vi "Teleop.vi"(10 "Match Info":T1={"Autonomous Elapsed Seconds"=0.0, "TeleOp Elapsed Seconds"=0.0, "Disabled Elapsed Seconds"=0.0, "Visited Autonomous"=FALSE, "Visited TeleOp"=FALSE, "Visited Disabled"=FALSE, "Autonomous Settings"={"Autonomous Style"=enum."Independent", "VI Refnum"=refnum}}, 11 "Call Context":T2) -> ()   [LabVIEW 2013]
doc: "This VI is called for each TeleOp packet received from the DS where the robot is not disabled. It is often used to read from the joysticks and update I/O or to update setpoints for timed control loops. It should complete and return within 20 milliseconds or it may miss DS packets."
uses:
  <vilib>/Rock Robotics/WPI/DriverStation/WPI_DriverStationDerivedRobotMode.ctl
  <vilib>/Rock Robotics/WPI/DriverStation/WPI_DriverStationMatch Info.ctl
  <vilib>/Rock Robotics/WPI/DriverStation/DriverStationLCD/WPI_DriverStationLCDLCDLine.ctl
  Robot Global Data.vi
  <vilib>/Rock Robotics/WPI/Joystick/WPI_JoystickGetSetRefNum.vi
  <vilib>/Rock Robotics/WPI/RobotDrive/WPI_RobotDriveGetSetRefNum.vi
  <vilib>/Rock Robotics/WPI/Solenoid/WPI_SolenoidSetEnum.vi
  <vilib>/Rock Robotics/WPI/Solenoid/WPI_SolenoidValue.ctl
panel:
  out "Numeric 1":dbl(slide) scale=0.0..100.0
  out "Boolean 2":bool
  out "Boolean 1":bool
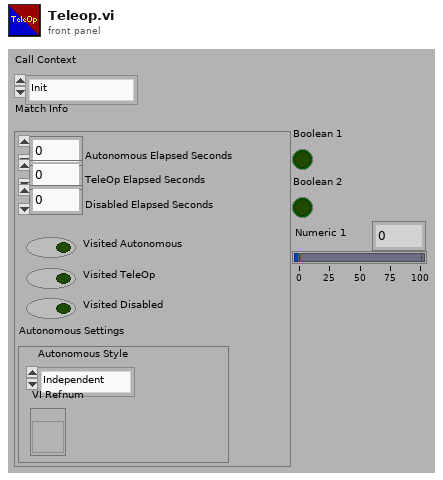
[diagram p1: front panel]
types:
  T1 = typedef "WPI_DriverStationMatch Info.ctl" = cluster{"Autonomous Elapsed Seconds":dbl, "TeleOp Elapsed Seconds":dbl, "Disabled Elapsed Seconds":dbl, "Visited Autonomous":bool, "Visited TeleOp":bool, "Visited Disabled":bool, "Autonomous Settings":cluster{"Autonomous Style":enum16{"Iterative", "Independent"}, "VI Refnum":refnum<vi>}}
  T2 = typedef "WPI_DriverStationDerivedRobotMode.ctl" = enum16{"Init", "Execute", "Stop"}
  T3 = typedef "WPI_DriverStationLCDLCDLine.ctl" = enum16{"Main - Line 1", "User - Line 2", "User - Line 3", "User - Line 4", "User - Line 5", "User - Line 6"}
  T4 = typedef "WPI_JoystickDevRef.ctl" = cluster{"Device":T5}
  T5 = typedef "WPI_JoystickDeviceEnum.ctl" = enum16{"USB 1", "USB 2", "USB 3", "USB 4", "Kinect 1", "Kinect 2"}
  T6 = typedef "WPI_JoystickButtonState.ctl" = cluster{"Button 1":bool, "Button 2":bool, "Button 3":bool, "Button 4":bool, "Button 5":bool, "Button 6":bool, "Button 7":bool, "Button 8":bool, "Button 9":bool, "Button 10":bool, "Button 11":bool, "Button 12":bool}
  T7 = cluster{"axis 1 (x)":dbl, "axis 2 (y)":dbl, "axis 3 (throttle)":dbl, "axis 4":dbl, "axis 5":dbl, "axis 6":dbl}
  T8 = typedef "WPI_SolenoidValue.ctl" = enum16{"Off", "On", "Forward", "Reverse"}
  T9 = typedef "WPI_SolenoidDevRef.ctl" = cluster{"DevStatus":errorcluster, "Solenoid Module":T10, "Forward Solenoid Channel":T11, "Reverse Solenoid Channel":T11}
  T10 = typedef "FPGA_TypedefSolenoidModule.ctl" = enum16{"Solenoid Module 1", "Solenoid Module 2"}
  T11 = typedef "WPI_SolenoidChannel.ctl" = enum8{"Solenoid 1", "Solenoid 2", "Solenoid 3", "Solenoid 4", "Solenoid 5", "Solenoid 6", "Solenoid 7", "Solenoid 8", "Invalid"}
  T12 = typedef "WPI_RobotDriveDevRef.ctl" = cluster{"DevStatus":errorcluster, "Motors[]":T13[], "Square Inputs":bool, "Max Output":dbl, "Isochronous":bool}
  T13 = typedef "WPI_MotorControlDeviceRef.ctl" = cluster{"DeviceStatus":errorcluster, "Type":enum16{"PWM", "CAN"}, "PWM":cluster{"Digital Module":T14, "PWM Channel":T15, "DeadBand":T16}, "CAN":cluster{"Device Number":u8, "Control Mode":T17, "Semaphore":T18, "Max Vout":dbl}, "Invert":bool, "TransformRef":T19, "InvTransformRef":T19}
  T14 = typedef "FPGA_TypedefDigitalModule.ctl" = enum16{"Digital Module 1", "Digital Module 2"}
  T15 = typedef "FPGA_DIOPWMChannel.ctl" = enum8{"PWM 1", "PWM 2", "PWM 3", "PWM 4", "PWM 5", "PWM 6", "PWM 7", "PWM 8", "PWM 9", "PWM 10", "Invalid"}
  T16 = typedef "WPI_PWMDeadband.ctl" = cluster{"Name":string, "maxPositivePwm":i32, "minPositivePwm":i32, "centerPwm":i32, "maxNegativePwm":i32, "minNegativePwm":i32, "angularRange":u16}
  T17 = typedef "WPI_CANJaguar_ControlMode.ctl" = enum8{"Percent VBus", "Current", "Speed", "Position", "Voltage"}
  T18 = typedef "Semaphore RefNum" = refnum<k1>
  T19 = typedef "WPI_PWMTransform_ConPane.ctl" = refnum<vi>
  T20 = enum16{"Reset", "Start", "Reset 2", "Manual", "Get ready to Fire", "Disengage Gearbox", "Ready to Fire", "Firing", "Firing Completed", "Reengage Gearbox"}
  T21 = typedef "WPI_AnalogChannelDevRef.ctl" = cluster{"DevStatus":errorcluster, "Analog Module":T22, "Analog Channel":T23}
  T22 = typedef "FPGA_TypedefAnalogModule.ctl" = enum16{"Analog Module 1", "Analog Module 2"}
  T23 = typedef "FPGA_AIChannel.ctl" = enum8{"AI 1", "AI 2", "AI 3", "AI 4", "AI 5", "AI 6", "AI 7", "AI 8", "Invalid"}
  T24 = typedef "WPI_DigitalInputDevRef.ctl" = cluster{"DevStatus":errorcluster, "DIO Channel":T25, "Digital Module":T14}
  T25 = typedef "FPGA_DIOChannel.ctl" = enum8{"DIO 1", "DIO 2", "DIO 3", "DIO 4", "DIO 5", "DIO 6", "DIO 7", "DIO 8", "DIO 9", "DIO 10", "DIO 11", "DIO 12", "DIO 13", "DIO 14", "Invalid"}
  T26 = typedef "WPI_RelayDevRef.ctl" = cluster{"DevStatus":errorcluster, "Relay Channel":T27, "Digital Module":T14, "Relay Direction":T28}
  T27 = typedef "FPGA_DIORelayChannel.ctl" = enum8{"Relay 1", "Relay 2", "Relay 3", "Relay 4", "Relay 5", "Relay 6", "Relay 7", "Relay 8", "Invalid"}
  T28 = typedef "WPI_RelayDirection.ctl" = enum16{"Both directions", "Forward only", "Reverse only"}
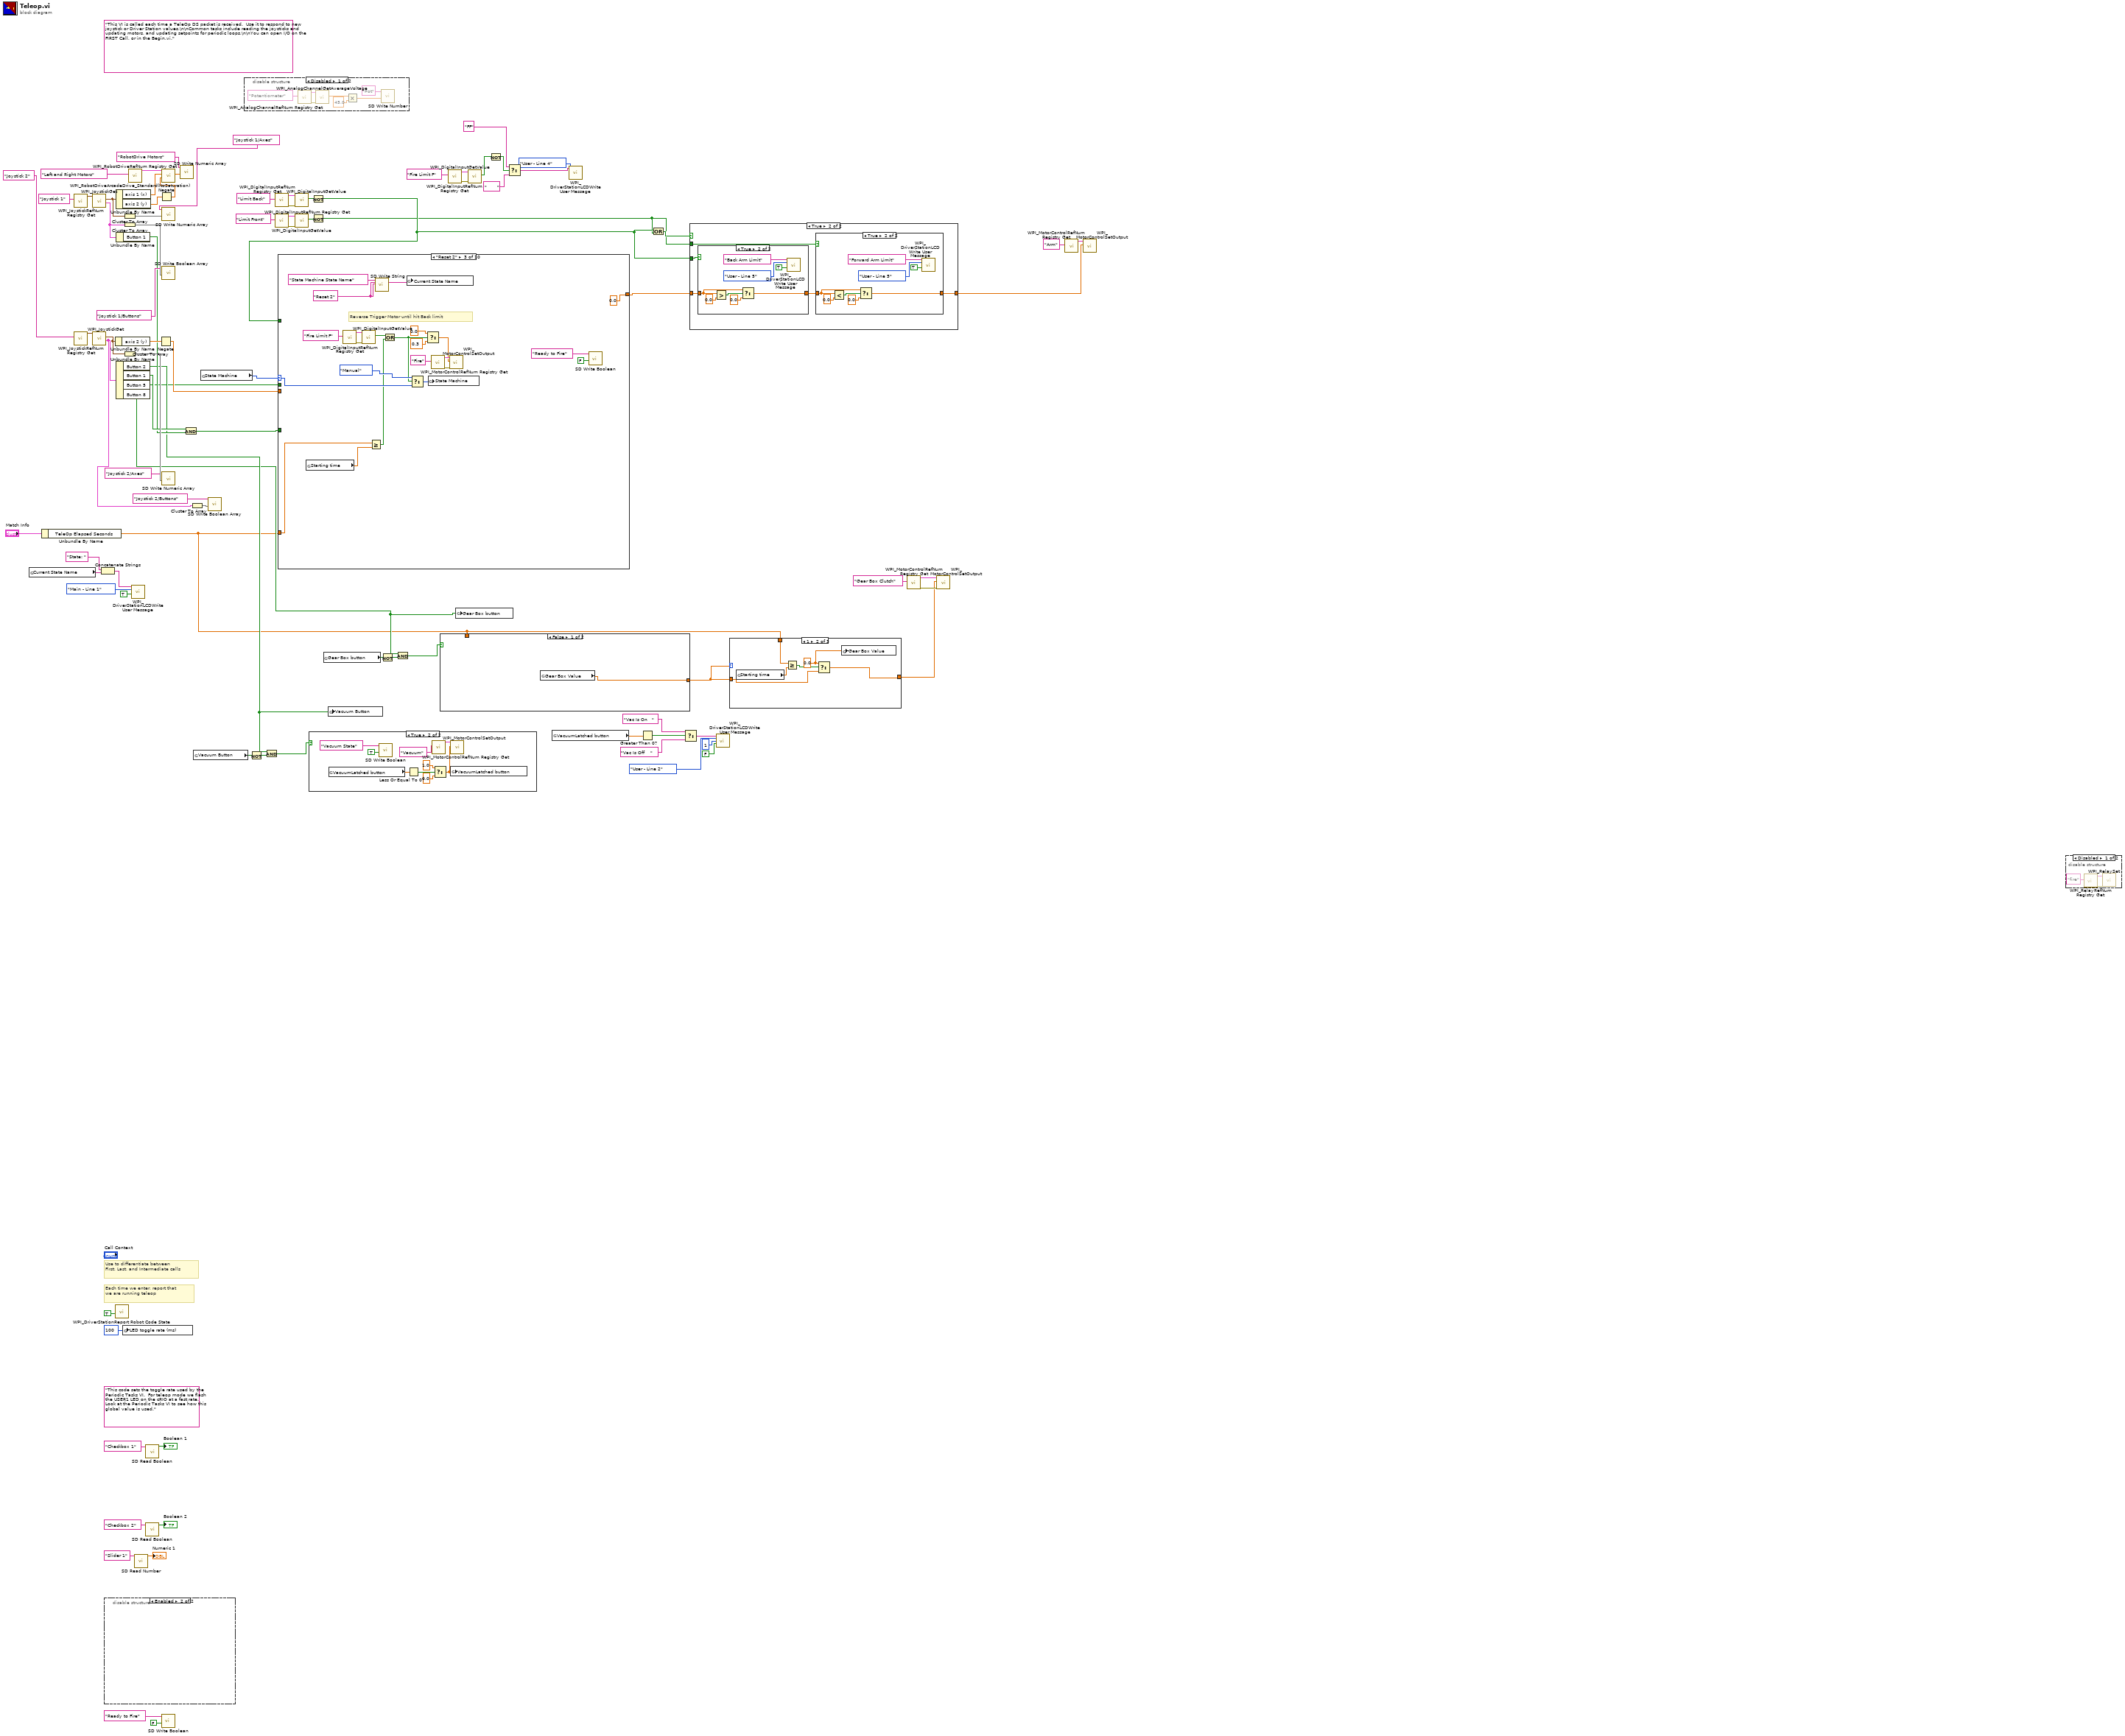
[diagram p0: block diagram]
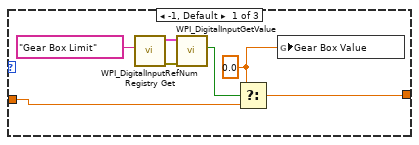
[diagram p2: hidden frame]
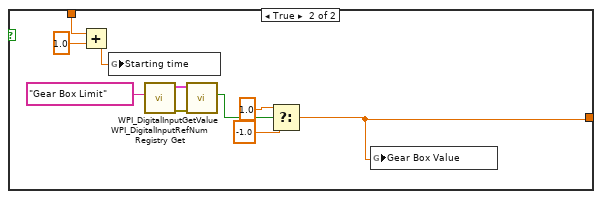
[diagram p4: hidden frame]
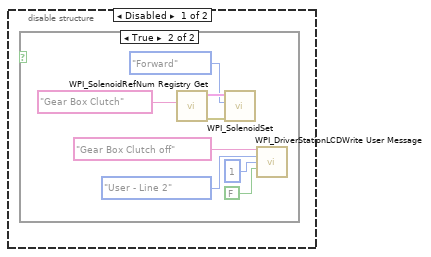
[diagram p11: hidden frame]
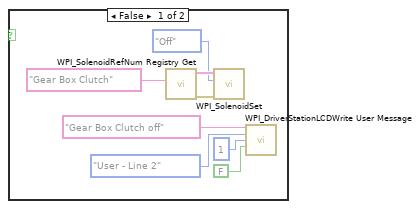
[diagram p12: hidden frame]
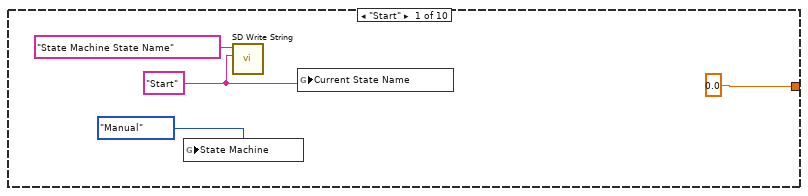
[diagram p13: hidden frame]
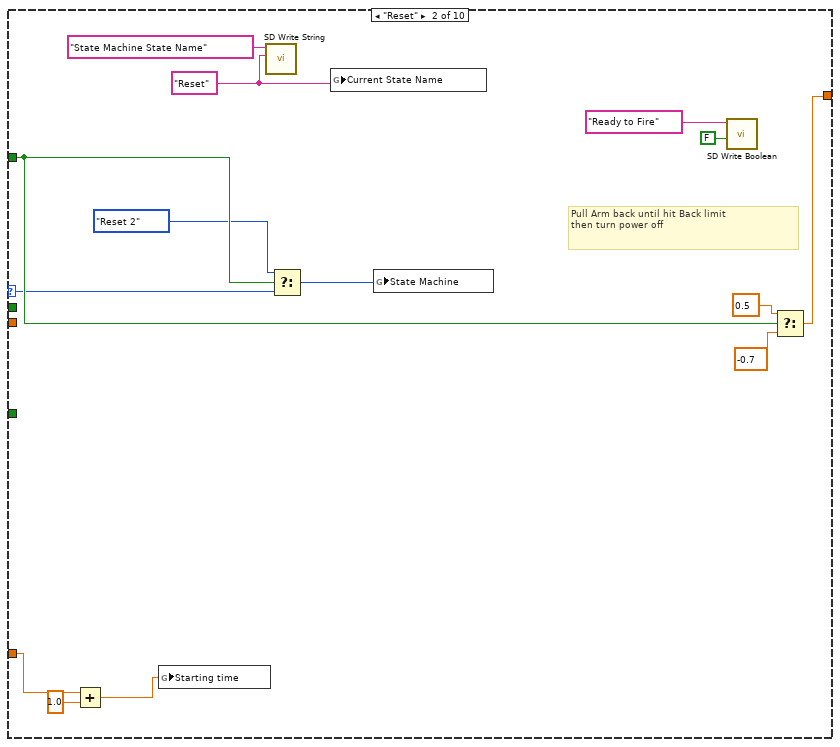
[diagram p14: hidden frame]
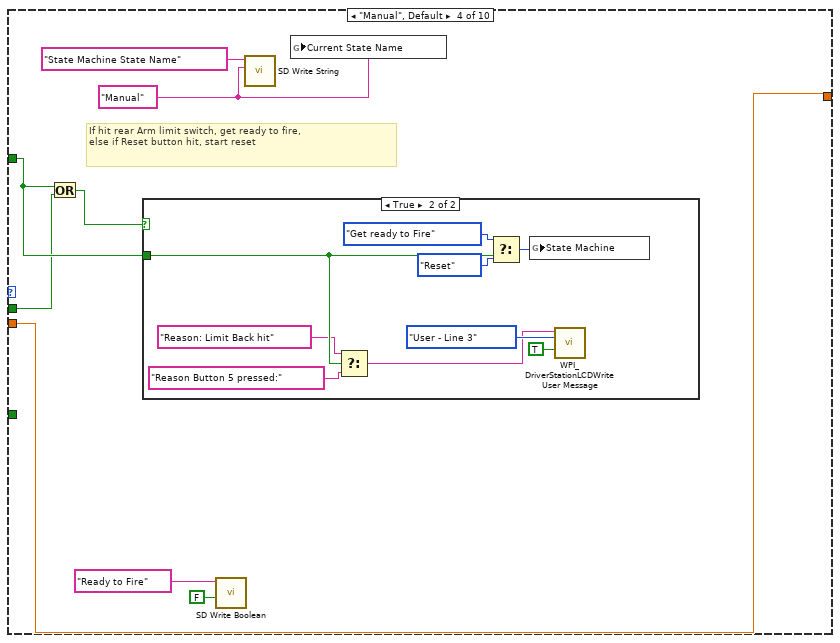
[diagram p15: hidden frame]
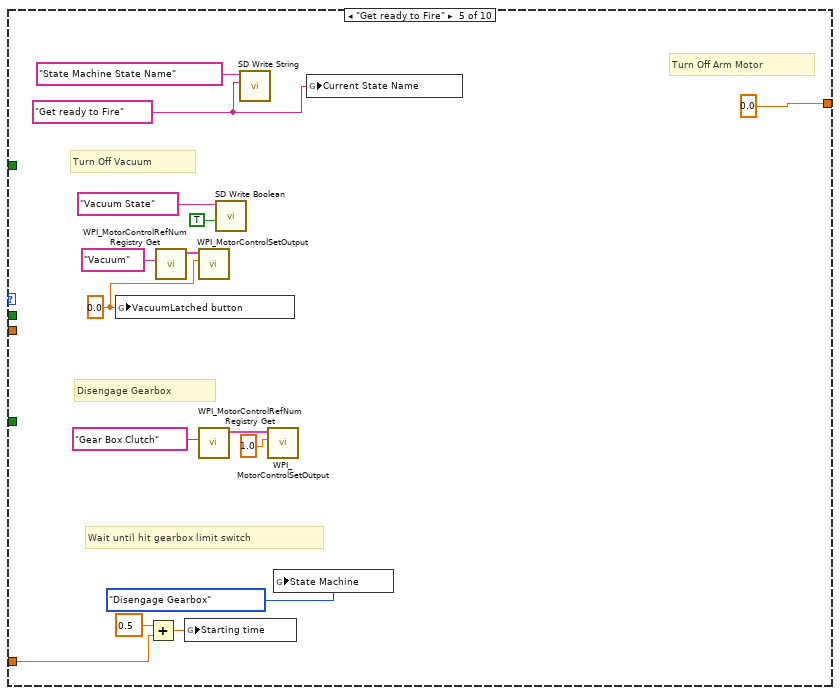
[diagram p17: hidden frame]
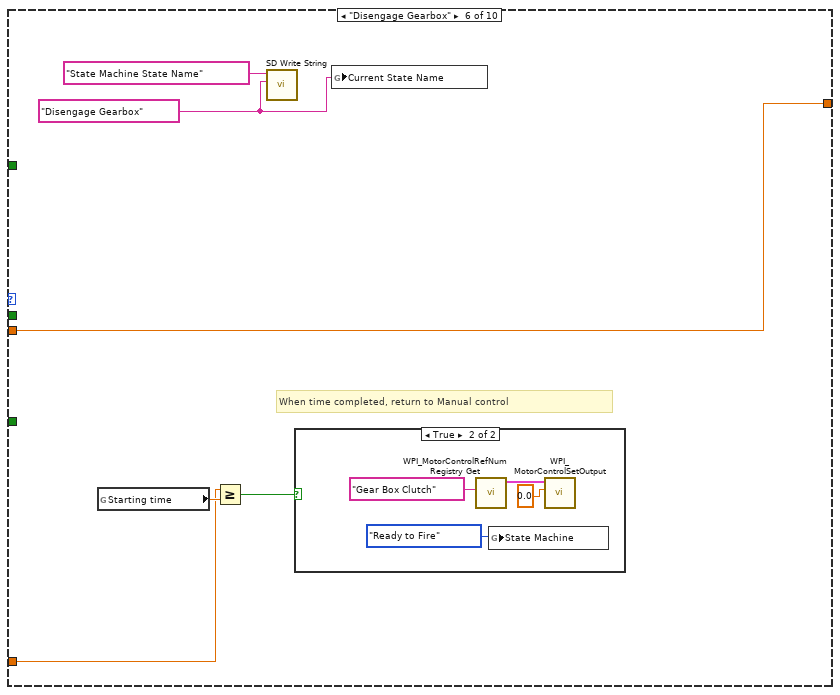
[diagram p18: hidden frame]
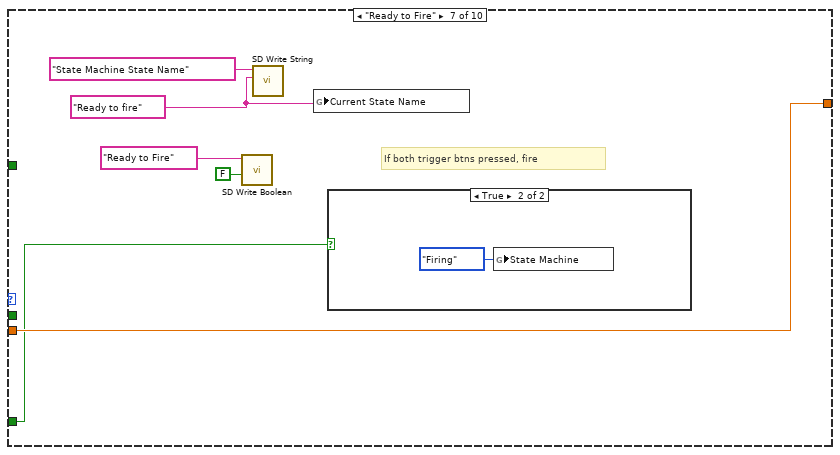
[diagram p20: hidden frame]
diagram:
  (unwired) "This code sets the toggle rate used by the Periodic Tasks VI.  For teleop mode we flash the USER1 LED on the cRIO at a fast rate.  Look at the Periodic Tasks VI to see how this global value is used."
  (unwired) "This VI is called each time a TeleOp DS packet is received.  Use it to respond to new joystick or Driver Station values.\n\nCommon tasks include reading the joysticks and updating motors, and updating setpoints for periodic loops.\n\nYou can open I/O on the FIRST Call, or in the Begin.vi."
  # "Each time we enter, report that\nwe are running teleop"
  # "Use to differentiate between\nFirst, Last, and Intermediate calls"
  n1 = global read "Robot Global Data.vi" "Current State Name"() -> (w23:string)
  n2 = Unbundle By Name("Match Info") -> ("TeleOp Elapsed Seconds"=w1:dbl)
  n3 = call <vilib>:"WPI_JoystickRefNum Registry Get.vi"("refnum name"="Joystick 1") -> ("JoystickDevRef"=w87:T4)  [unwired: 1 in, 9 out]
  n4 = call <vilib>:"WPI_JoystickRefNum Registry Get.vi"("refnum name"="Joystick 2") -> ("JoystickDevRef"=w70:T4)  [unwired: 1 in, 9 out]
  n5 = call <vilib>:"WPI_JoystickGet.vi"("JoystickDevRef"=w87) -> ("Buttons"=w62:T6, "Axes"=w82:T7)  [unwired: 1 in, 4 out]
  n6 = call <vilib>:"WPI_JoystickGet.vi"("JoystickDevRef"=w70) -> ("Buttons"=w64:T6, "Axes"=w67:T7)  [unwired: 1 in, 4 out]
  n7 = Concatenate Strings("State: " ("line text"), w23) -> (w22:string)
  n8 = disable-structure shown="Enabled" {
    frame Disabled {
      n9 = case shown="True" {
        selector: _ -> [_ _]
        frame False {
          n10 = call <vilib>:"WPI_SolenoidRefNum Registry Get.vi"("refnum name"="Gear Box Clutch") -> ("error out"=w98:errorcluster, "SolenoidDevRef"=w99:T9)  [unwired: 9 in]
          n11 = call-poly <vilib>:"WPI_SolenoidSet.vi"("error in (no error)"=w98, "Value"=WPI_SolenoidValue."Off", "SolenoidDevRef"=w99) -> ()  [unwired: 7 in, 2 out]
          n12 = call <vilib>:"WPI_DriverStationLCDWrite User Message.vi"("line text"="Gear Box Clutch off", "line"=WPI_DriverStationLCDLCDLine."User - Line 2", "starting column"=i8 1, "clear line before write (T)"=FALSE) -> ()  [unwired: 11 in, 1 out]
        }
        frame True {
          n13 = call <vilib>:"WPI_SolenoidRefNum Registry Get.vi"("refnum name"="Gear Box Clutch") -> ("error out"=w106:errorcluster, "SolenoidDevRef"=w107:T9)  [unwired: 9 in]
          n14 = call-poly <vilib>:"WPI_SolenoidSet.vi"("error in (no error)"=w106, "Value"=WPI_SolenoidValue."Forward", "SolenoidDevRef"=w107) -> ()  [unwired: 7 in, 2 out]
          n15 = call <vilib>:"WPI_DriverStationLCDWrite User Message.vi"("line text"="Gear Box Clutch off", "line"=WPI_DriverStationLCDLCDLine."User - Line 2", "starting column"=i8 1, "clear line before write (T)"=FALSE) -> ()  [unwired: 11 in, 1 out]
        }
      }
    }
    frame Enabled {
    }
  }
  n16 = Unbundle By Name(w67) -> ("axis 2 (y)"=w63:dbl)
  n17 = call <vilib>:"WPI_DriverStationReport Robot Code State.vi"("TeleOp"=TRUE ("Autonomous")) -> ()  [unwired: 10 in, 1 out]
  n18 = Unbundle By Name(w82) -> ("axis 1 (x)"=w89:dbl, "axis 2 (y)"=w12:dbl)
  n19 = Unbundle By Name(w62) -> ("Button 1"=w60:bool)
  n20 = Unbundle By Name(w64) -> ("Button 2"=w45:bool, "Button 1"=w61:bool, "Button 5"=w27:bool, "Button 8"=w4:bool)
  n21 = global write "Robot Global Data.vi" "LED toggle rate (ms)"(u32 100 ("LED ms toggle rate")) -> ()
  n22 = Cluster To Array(cluster=w82) -> (array=w81:dbl[])
  n23 = Cluster To Array(cluster=w62) -> (array=w84:bool[])
  n24 = Cluster To Array(cluster=w67) -> (array=w66:dbl[])
  n25 = call <vilib>:"WPI_RobotDriveRefNum Registry Get.vi"("refnum name"="Left and Right Motors") -> ("RobotDriveDevRef"=w90:T12)  [unwired: 1 in, 9 out]
  n26 = call <vilib>:"WPI_DriverStationLCDWrite User Message.vi"("line text"=w22, "line"=WPI_DriverStationLCDLCDLine."Main - Line 1", "clear line before write (T)"=TRUE) -> ()  [unwired: 12 in, 1 out]
  n27 = call <vilib>:"SD Read Number.vi"("Name"="Slider 1" ("refnum name")) -> ("Numeric"=→"Numeric 1":dbl)  [unwired: 8 in, 2 out]
  n28 = call <vilib>:"SD Read Boolean.vi"("Name"="Checkbox 1" ("refnum name")) -> ("Boolean"=→"Boolean 1":bool)  [unwired: 8 in, 2 out]
  n29 = call <vilib>:"SD Read Boolean.vi"("Name"="Checkbox 2" ("refnum name")) -> ("Boolean"=→"Boolean 2":bool)  [unwired: 8 in, 2 out]
  n30 = Negate(x=w63) -> (-x=w48:dbl)
  n31 = Negate(x=w12) -> (-x=w11:dbl)
  n32 = call <vilib>:"SD Write Boolean.vi"("Boolean"=FALSE, "Name"="Ready to Fire") -> ()  [unwired: 8 in, 2 out]
  n33 = call <vilib>:"WPI_RobotDriveArcadeDrive_Standard(NoSaturation).vi"("Y axis value"=w11, "X axis value"=w89, "RobotDriveDevRef"=w90) -> ("Motor Values"=w78:dbl[])  [unwired: 1 in, 7 out]
  n34 = call <vilib>:"SD Write Numeric Array.vi"("Numeric Array"=w81, "Name"="Joystick 1/Axes") -> ()  [unwired: 8 in, 2 out]
  n35 = call <vilib>:"SD Write Boolean Array.vi"("Boolean Array"=w84, "Name"="Joystick 1/Buttons") -> ()  [unwired: 8 in, 2 out]
  n36 = call <vilib>:"SD Write Numeric Array.vi"("Numeric Array"=w66, "Name"="Joystick 2/Axes") -> ()  [unwired: 8 in, 2 out]
  n37 = call <vilib>:"SD Write Numeric Array.vi"("Numeric Array"=w78, "Name"="RobotDrive Motors") -> ()  [unwired: 8 in, 2 out]
  n38 = And(x=w61, y=w60) -> (x .and. y?=w43:bool)
  n39 = Cluster To Array(cluster=w64) -> (array=w69:bool[])
  n40 = global read "Robot Global Data.vi" "Vacuum Button"() -> (w46:bool)
  n41 = global read "Robot Global Data.vi" "State Machine"() -> (w44:T20)
  n42 = call <vilib>:"SD Write Boolean Array.vi"("Boolean Array"=w69, "Name"="Joystick 2/Buttons") -> ()  [unwired: 8 in, 2 out]
  n43 = disable-structure shown="Disabled" {
    frame Disabled {
      n44 = call <vilib>:"WPI_AnalogChannelRefNum Registry Get.vi"("refnum name"="Potentiometer") -> ("error out"=w115:errorcluster, "AIDeviceRef"=w114:T21)  [unwired: 9 in]
      n45 = call <vilib>:"WPI_AnalogChannelGetAverageVoltage.vi"("error in (no error)"=w115, "AIDeviceRef"=w114) -> ("Voltage"=w110:dbl)  [unwired: 7 in, 2 out]
      n46 = Multiply(x=w110, y=45.0) -> (x*y=w109:dbl)
      n47 = call <vilib>:"SD Write Number.vi"("Numeric"=w109, "Name"="Pot") -> ()  [unwired: 8 in, 2 out]
    }
    frame Enabled {
    }
  }
  n48 = Not(x=w46) -> (.not. x?=w47:bool)
  n49 = And(x=w45, y=w47) -> (x .and. y?=w37:bool)
  n50 = call <vilib>:"WPI_DigitalInputRefNum Registry Get.vi"("refnum name"="Limit Back") -> ("error out"=w54:errorcluster, "DigitalInputDevRef"=w53:T24)  [unwired: 9 in]
  n51 = call <vilib>:"WPI_DigitalInputRefNum Registry Get.vi"("refnum name"="Limit Front") -> ("error out"=w51:errorcluster, "DigitalInputDevRef"=w52:T24)  [unwired: 9 in]
  n52 = call <vilib>:"WPI_DigitalInputGetValue.vi"("error in (no error)"=w54, "DigitalInputDevRef"=w53) -> ("Value"=w42:bool)  [unwired: 7 in, 2 out]
  n53 = call <vilib>:"WPI_DigitalInputGetValue.vi"("error in (no error)"=w51, "DigitalInputDevRef"=w52) -> ("Value"=w40:bool)  [unwired: 7 in, 2 out]
  n54 = case shown="True" w37 {
    frame False {
    }
    frame True {
      n55 = global read "Robot Global Data.vi" "VacuumLatched button"() -> (w122:dbl)
      n56 = call <vilib>:"SD Write Boolean.vi"("Boolean"=TRUE, "Name"="Vacuum State") -> ()  [unwired: 8 in, 2 out]
      n57 = Less Or Equal To 0?(x=w122) -> (x <= 0?=w117:bool)
      n58 = call <vilib>:"WPI_MotorControlRefNum Registry Get.vi"("refnum name"="Vacuum") -> ("MotorControlDevRef"=w119:T13)  [unwired: 9 in, 1 out]
      n59 = Select(t=1.0 ("Numeric"), s=w117, f=0.0) -> (s? t:f=w118:dbl)
      n60 = call <vilib>:"WPI_MotorControlSetOutput.vi"("Output"=w118, "MotorControlDevRef"=w119) -> ()  [unwired: 7 in, 3 out]
      n61 = global write "Robot Global Data.vi" "VacuumLatched button"(w118) -> ()
    }
  }
  n62 = Not(x=w42) -> (.not. x?=w41:bool)
  n63 = case shown="\"Reset 2\"" w44 {
    selector: w44 -> [_ w136 w157 _ _ _ _ w218 _ _]
    tunnel: w48 -> [_ _ _ w166 _ w202 w212 w230 w239 w246]
    tunnel: [0.0 w137 0.0 w166 0.0 w202 w212 w230 w239 w246] -> w38
    tunnel: w43 -> [_ _ _ _ _ _ w208 _ _ _]
    tunnel: w41 -> [_ w140 _ w168 _ _ _ _ _ _]
    tunnel: w1 -> [_ w131 w146 _ w183 w197 _ _ _ _]
    tunnel: w27 -> [_ _ _ w165 _ _ _ _ _ _]
    frame "Start" {
      w126 = "Start" ("line text")
      n64 = global write "Robot Global Data.vi" "State Machine"(T20."Manual" ("State Machine")) -> ()
      n65 = call <vilib>:"SD Write String.vi"("Table Prefix"=w126, "Name"="State Machine State Name") -> ()  [unwired: 8 in, 2 out]
      n66 = global write "Robot Global Data.vi" "Current State Name"(w126) -> ()
    }
    frame "Reset" {
      w134 = "Reset" ("line text")
      # "Pull Arm back until hit Back limit\nthen turn power off"
      n67 = Add(x=w131, y=1.0) -> (x+y=w129:dbl)
      n68 = global write "Robot Global Data.vi" "Starting time"(w129) -> ()
      n69 = call <vilib>:"SD Write String.vi"("Table Prefix"=w134, "Name"="State Machine State Name") -> ()  [unwired: 8 in, 2 out]
      n70 = Select(t=T20."Reset 2" ("s? t:f"), s=w140, f=w136) -> (s? t:f=w133:T20)
      n71 = global write "Robot Global Data.vi" "Current State Name"(w134) -> ()
      n72 = global write "Robot Global Data.vi" "State Machine"(w133) -> ()
      n73 = call <vilib>:"SD Write Boolean.vi"("Boolean"=FALSE, "Name"="Ready to Fire") -> ()  [unwired: 8 in, 2 out]
      n74 = Select(t=0.5, s=w140, f=-0.7) -> (s? t:f=w137:dbl)
    }
    frame "Reset 2" {
      w149 = "Reset 2" ("line text")
      # "Reverse Trigger Motor until hit Back limit"
      n75 = global read "Robot Global Data.vi" "Starting time"() -> (w145:dbl)
      n76 = call <vilib>:"WPI_DigitalInputRefNum Registry Get.vi"("refnum name"="Fire Limit F") -> ("error out"=w154:errorcluster, "DigitalInputDevRef"=w153:T24)  [unwired: 9 in]
      n77 = call <vilib>:"WPI_DigitalInputGetValue.vi"("error in (no error)"=w154, "DigitalInputDevRef"=w153) -> ("Value"=w147:bool)  [unwired: 7 in, 2 out]
      n78 = Greater Or Equal?(x=w146, y=w145) -> (x >= y?=w144:bool)
      n79 = call <vilib>:"SD Write String.vi"("Table Prefix"=w149, "Name"="State Machine State Name") -> ()  [unwired: 8 in, 2 out]
      n80 = Or(x=w147, y=w144) -> (x .or. y?=w143:bool)
      n81 = global write "Robot Global Data.vi" "Current State Name"(w149) -> ()
      n82 = Select(t=T20."Manual" ("s? t:f"), s=w143, f=w157) -> (s? t:f=w156:T20)
      n83 = Select(t=0.0, s=w143, f=0.3) -> (s? t:f=w151:dbl)
      n84 = global write "Robot Global Data.vi" "State Machine"(w156) -> ()
      n85 = call <vilib>:"WPI_MotorControlRefNum Registry Get.vi"("refnum name"="Fire") -> ("error out"=w162:errorcluster, "MotorControlDevRef"=w161:T13)  [unwired: 9 in]
      n86 = call <vilib>:"WPI_MotorControlSetOutput.vi"("error in (no error)"=w162, "Output"=w151, "MotorControlDevRef"=w161) -> ()  [unwired: 6 in, 3 out]
      n87 = call <vilib>:"SD Write Boolean.vi"("Boolean"=FALSE, "Name"="Ready to Fire") -> ()  [unwired: 8 in, 2 out]
    }
    frame "Manual", Default {
      w167 = "Manual" ("line text")
      # "If hit rear Arm limit switch, get ready to fire, \nelse if Reset button hit, start reset"
      n88 = Or(x=w168, y=w165) -> (x .or. y?=w169:bool)
      n89 = case shown="True" w169 {
        tunnel: w168 -> [_ w178]
        frame False {
        }
        frame True {
          n90 = Select(t="Reason: Limit Back hit" ("line text"), s=w178, f="Reason Button 5 pressed:" ("line text")) -> (s? t:f=w173:string)
          n91 = Select(t=T20."Get ready to Fire" ("State Machine"), s=w178, f=T20."Reset" ("State Machine")) -> (s? t:f=w180:T20)
          n92 = global write "Robot Global Data.vi" "State Machine"(w180) -> ()
          n93 = call <vilib>:"WPI_DriverStationLCDWrite User Message.vi"("line text"=w173, "line"=WPI_DriverStationLCDLCDLine."User - Line 3", "clear line before write (T)"=TRUE) -> ()  [unwired: 12 in, 1 out]
        }
      }
      n94 = call <vilib>:"SD Write Boolean.vi"("Boolean"=FALSE, "Name"="Ready to Fire") -> ()  [unwired: 8 in, 2 out]
      n95 = call <vilib>:"SD Write String.vi"("Table Prefix"=w167, "Name"="State Machine State Name") -> ()  [unwired: 8 in, 2 out]
      n96 = global write "Robot Global Data.vi" "Current State Name"(w167) -> ()
    }
    frame "Get ready to Fire" {
      w186 = "Get ready to Fire" ("line text")
      w192 = 0.0 ("f")
      # "Wait until hit gearbox limit switch"
      # "Disengage Gearbox"
      # "Turn Off Arm Motor"
      # "Turn Off Vacuum"
      n97 = global write "Robot Global Data.vi" "VacuumLatched button"(w192) -> ()
      n98 = Add(x=0.5 ("Starting time"), y=w183) -> (x+y=w184:dbl)
      n99 = call <vilib>:"WPI_MotorControlRefNum Registry Get.vi"("refnum name"="Vacuum") -> ("MotorControlDevRef"=w193:T13)  [unwired: 9 in, 1 out]
      n100 = global write "Robot Global Data.vi" "Starting time"(w184) -> ()
      n101 = call <vilib>:"WPI_MotorControlSetOutput.vi"("Output"=w192, "MotorControlDevRef"=w193) -> ()  [unwired: 7 in, 3 out]
      n102 = call <vilib>:"WPI_MotorControlRefNum Registry Get.vi"("refnum name"="Gear Box Clutch") -> ("MotorControlDevRef"=w191:T13)  [unwired: 9 in, 1 out]
      n103 = call <vilib>:"SD Write Boolean.vi"("Boolean"=TRUE, "Name"="Vacuum State") -> ()  [unwired: 8 in, 2 out]
      n104 = call <vilib>:"SD Write String.vi"("Table Prefix"=w186, "Name"="State Machine State Name") -> ()  [unwired: 8 in, 2 out]
      n105 = call <vilib>:"WPI_MotorControlSetOutput.vi"("Output"=1.0 ("Numeric"), "MotorControlDevRef"=w191) -> ()  [unwired: 7 in, 3 out]
      n106 = global write "Robot Global Data.vi" "State Machine"(T20."Disengage Gearbox" ("State Machine")) -> ()
      n107 = global write "Robot Global Data.vi" "Current State Name"(w186) -> ()
    }
    frame "Disengage Gearbox" {
      w200 = "Disengage Gearbox" ("line text")
      # "When time completed, return to Manual control"
      n108 = global read "Robot Global Data.vi" "Starting time"() -> (w199:dbl)
      n109 = Greater Or Equal?(x=w197, y=w199) -> (x >= y?=w198:bool)
      n110 = call <vilib>:"SD Write String.vi"("Table Prefix"=w200, "Name"="State Machine State Name") -> ()  [unwired: 8 in, 2 out]
      n111 = case shown="True" w198 {
        frame False {
        }
        frame True {
          n112 = call <vilib>:"WPI_MotorControlRefNum Registry Get.vi"("refnum name"="Gear Box Clutch") -> ("MotorControlDevRef"=w206:T13)  [unwired: 9 in, 1 out]
          n113 = global write "Robot Global Data.vi" "State Machine"(T20."Ready to Fire" ("State Machine")) -> ()
          n114 = call <vilib>:"WPI_MotorControlSetOutput.vi"("Output"=0.0 ("Numeric"), "MotorControlDevRef"=w206) -> ()  [unwired: 7 in, 3 out]
        }
      }
      n115 = global write "Robot Global Data.vi" "Current State Name"(w200) -> ()
    }
    frame "Ready to Fire" {
      w207 = "Ready to fire" ("line text")
      # "If both trigger btns pressed, fire"
      n116 = call <vilib>:"SD Write Boolean.vi"("Boolean"=FALSE, "Name"="Ready to Fire") -> ()  [unwired: 8 in, 2 out]
      n117 = call <vilib>:"SD Write String.vi"("Table Prefix"=w207, "Name"="State Machine State Name") -> ()  [unwired: 8 in, 2 out]
      n118 = global write "Robot Global Data.vi" "Current State Name"(w207) -> ()
      n119 = case shown="True" w208 {
        frame False {
        }
        frame True {
          n120 = global write "Robot Global Data.vi" "State Machine"(T20."Firing" ("State Machine")) -> ()
        }
      }
    }
    frame "Firing" {
      w215 = "Firing" ("line text")
      # "Run Trigger motor forward until hit forward limit"
      n121 = call <vilib>:"WPI_DigitalInputRefNum Registry Get.vi"("refnum name"="Fire Limit F") -> ("error out"=w221:errorcluster, "DigitalInputDevRef"=w222:T24)  [unwired: 9 in]
      n122 = call <vilib>:"WPI_DigitalInputGetValue.vi"("error in (no error)"=w221, "DigitalInputDevRef"=w222) -> ("Value"=w220:bool)  [unwired: 7 in, 2 out]
      n123 = Not(x=w220) -> (.not. x?=w217:bool)
      n124 = call <vilib>:"SD Write String.vi"("Table Prefix"=w215, "Name"="State Machine State Name") -> ()  [unwired: 8 in, 2 out]
      n125 = Select(t=T20."Firing Completed" ("s? t:f"), s=w217, f=w218) -> (s? t:f=w216:T20)
      n126 = global write "Robot Global Data.vi" "Current State Name"(w215) -> ()
      n127 = global write "Robot Global Data.vi" "State Machine"(w216) -> ()
      n128 = Select(t=0.0, s=w217, f=-0.8) -> (s? t:f=w224:dbl)
      n129 = call <vilib>:"WPI_MotorControlRefNum Registry Get.vi"("refnum name"="Fire") -> ("error out"=w229:errorcluster, "MotorControlDevRef"=w228:T13)  [unwired: 9 in]
      n130 = call <vilib>:"WPI_MotorControlSetOutput.vi"("error in (no error)"=w229, "Output"=w224, "MotorControlDevRef"=w228) -> ()  [unwired: 6 in, 3 out]
    }
    frame "Firing Completed" {
      w232 = "Firing Completed" ("line text")
      # "Run for .5 secs"
      # "Re-engage Gearbox by running clutch motor in reverse"
      # "Turn off Trigger motor"
      n131 = call <vilib>:"WPI_MotorControlRefNum Registry Get.vi"("refnum name"="Fire") -> ("error out"=w238:errorcluster, "MotorControlDevRef"=w237:T13)  [unwired: 9 in]
      n132 = call <vilib>:"WPI_MotorControlSetOutput.vi"("error in (no error)"=w238, "Output"=0.0, "MotorControlDevRef"=w237) -> ()  [unwired: 6 in, 3 out]
      n133 = call <vilib>:"SD Write String.vi"("Table Prefix"=w232, "Name"="State Machine State Name") -> ()  [unwired: 8 in, 2 out]
      n134 = global write "Robot Global Data.vi" "State Machine"(T20."Reengage Gearbox" ("State Machine")) -> ()
      n135 = global write "Robot Global Data.vi" "Gear Box Value"(-1.0 ("Numeric")) -> ()
      n136 = global write "Robot Global Data.vi" "Current State Name"(w232) -> ()
    }
    frame "Reengage Gearbox" {
      w244 = "Reengage Gearbox" ("line text")
      # "Keep moving gearbox motor until hit limit switch"
      n137 = call <vilib>:"WPI_DigitalInputRefNum Registry Get.vi"("refnum name"="Gear Box Limit") -> ("error out"=w242:errorcluster, "DigitalInputDevRef"=w243:T24)  [unwired: 9 in]
      n138 = call <vilib>:"WPI_DigitalInputGetValue.vi"("error in (no error)"=w242, "DigitalInputDevRef"=w243) -> ("Value"=w240:bool)  [unwired: 7 in, 2 out]
      n139 = call <vilib>:"SD Write String.vi"("Table Prefix"=w244, "Name"="State Machine State Name") -> ()  [unwired: 8 in, 2 out]
      n140 = case shown="True" w240 {
        frame False {
        }
        frame True {
          n141 = global write "Robot Global Data.vi" "State Machine"(T20."Manual" ("State Machine")) -> ()
          n142 = call <vilib>:"WPI_MotorControlRefNum Registry Get.vi"("refnum name"="Gear Box Clutch") -> ("error out"=w247:errorcluster, "MotorControlDevRef"=w251:T13)  [unwired: 9 in]
          n143 = call <vilib>:"WPI_MotorControlSetOutput.vi"("error in (no error)"=w247, "Output"=0.0 ("Numeric"), "MotorControlDevRef"=w251) -> ()  [unwired: 6 in, 3 out]
        }
      }
      n144 = global write "Robot Global Data.vi" "Current State Name"(w244) -> ()
    }
  }
  n145 = Not(x=w40) -> (.not. x?=w39:bool)
  n146 = global read "Robot Global Data.vi" "Gear Box button"() -> (w6:bool)
  n147 = global write "Robot Global Data.vi" "Vacuum Button"(w45) -> ()
  n148 = Not(x=w6) -> (.not. x?=w7:bool)
  n149 = And(x=w4, y=w7) -> (x .and. y?=w5:bool)
  n150 = case shown="False" w5 {
    tunnel: w1 -> [_ w257]
    tunnel: [w252 w253] -> w2
    frame False {
      n151 = global read "Robot Global Data.vi" "Gear Box Value"() -> (w252:dbl)
    }
    frame True {
      n152 = Add(x=w257, y=1.0) -> (x+y=w261:dbl)
      n153 = global write "Robot Global Data.vi" "Starting time"(w261) -> ()
      n154 = call <vilib>:"WPI_DigitalInputRefNum Registry Get.vi"("refnum name"="Gear Box Limit") -> ("error out"=w259:errorcluster, "DigitalInputDevRef"=w260:T24)  [unwired: 9 in]
      n155 = call <vilib>:"WPI_DigitalInputGetValue.vi"("error in (no error)"=w259, "DigitalInputDevRef"=w260) -> ("Value"=w254:bool)  [unwired: 7 in, 2 out]
      n156 = Select(t=1.0, s=w254, f=-1.0) -> (s? t:f=w253:dbl)
      n157 = global write "Robot Global Data.vi" "Gear Box Value"(w253) -> ()
    }
  }
  n158 = call <vilib>:"WPI_DigitalInputRefNum Registry Get.vi"("refnum name"="Fire Limit F") -> ("error out"=w20:errorcluster, "DigitalInputDevRef"=w21:T24)  [unwired: 9 in]
  n159 = global write "Robot Global Data.vi" "Gear Box button"(w4) -> ()
  n160 = call <vilib>:"WPI_DigitalInputGetValue.vi"("error in (no error)"=w20, "DigitalInputDevRef"=w21) -> ("Value"=w14:bool)  [unwired: 7 in, 2 out]
  n161 = Not(x=w14) -> (.not. x?=w13:bool)
  n162 = Select(t="FF", s=w13, f="       ") -> (s? t:f=w17:string)
  n163 = global read "Robot Global Data.vi" "VacuumLatched button"() -> (w28:dbl)
  n164 = call <vilib>:"WPI_DriverStationLCDWrite User Message.vi"("line text"=w17, "line"=WPI_DriverStationLCDLCDLine."User - Line 4") -> ()  [unwired: 13 in, 1 out]
  n165 = Greater Than 0?(x=w28) -> (x > 0?=w29:bool)
  n166 = Or(x=w41, y=w39) -> (x .or. y?=w49:bool)
  n167 = Select(t="Vac Is On   ", s=w29, f="Vac Is Off    ") -> (s? t:f=w35:string)
  n168 = case shown="True" w49 {
    tunnel: w38 -> [w263 w268]
    tunnel: [w263 w266] -> w36
    tunnel: w41 -> [_ w265]
    tunnel: w39 -> [_ w264]
    frame False {
    }
    frame True {
      n169 = case shown="True" w265 {
        tunnel: w268 -> [w278 w284]
        tunnel: [w278 w286] -> w267
        frame False {
        }
        frame True {
          n170 = Greater?(x=w284, y=0.0) -> (0:w282:bool)
          n171 = Select(t=w284, s=w282, f=0.0) -> (s? t:f=w286:dbl)
          n172 = call <vilib>:"WPI_DriverStationLCDWrite User Message.vi"("line text"="Back Arm Limit", "line"=WPI_DriverStationLCDLCDLine."User - Line 5", "clear line before write (T)"=TRUE) -> ()  [unwired: 12 in, 1 out]
        }
      }
      n173 = case shown="True" w264 {
        tunnel: w267 -> [w269 w275]
        tunnel: [w269 w277] -> w266
        frame False {
        }
        frame True {
          n174 = Less?(x=w275, y=0.0) -> (x < y?=w273:bool)
          n175 = Select(t=w275, s=w273, f=0.0) -> (s? t:f=w277:dbl)
          n176 = call <vilib>:"WPI_DriverStationLCDWrite User Message.vi"("line text"="Forward Arm Limit", "line"=WPI_DriverStationLCDLCDLine."User - Line 5", "clear line before write (T)"=TRUE) -> ()  [unwired: 12 in, 1 out]
        }
      }
    }
  }
  n177 = call <vilib>:"WPI_DriverStationLCDWrite User Message.vi"("line text"=w35, "line"=WPI_DriverStationLCDLCDLine."User - Line 2", "starting column"=i8 1, "clear line before write (T)"=FALSE) -> ()  [unwired: 11 in, 1 out]
  n178 = case shown="1" w2 {
    tunnel: [w289 w295 w300] -> w3
    tunnel: w2 -> [w288 w296 w300]
    tunnel: w1 -> [_ w299 _]
    frame -1, Default {
      w287 = 0.0 ("t")
      n179 = call <vilib>:"WPI_DigitalInputRefNum Registry Get.vi"("refnum name"="Gear Box Limit") -> ("error out"=w292:errorcluster, "DigitalInputDevRef"=w293:T24)  [unwired: 9 in]
      n180 = call <vilib>:"WPI_DigitalInputGetValue.vi"("error in (no error)"=w292, "DigitalInputDevRef"=w293) -> ("Value"=w290:bool)  [unwired: 7 in, 2 out]
      n181 = Select(t=w287, s=w290, f=w288) -> (s? t:f=w289:dbl)
      n182 = global write "Robot Global Data.vi" "Gear Box Value"(w287) -> ()
    }
    frame 1 {
      w294 = 0.0 ("t")
      n183 = global read "Robot Global Data.vi" "Starting time"() -> (w298:dbl)
      n184 = Greater Or Equal?(x=w299, y=w298) -> (x >= y?=w297:bool)
      n185 = Select(t=w294, s=w297, f=w296) -> (s? t:f=w295:dbl)
      n186 = global write "Robot Global Data.vi" "Gear Box Value"(w294) -> ()
    }
    frame 0 {
    }
  }
  n187 = call <vilib>:"WPI_MotorControlRefNum Registry Get.vi"("refnum name"="Gear Box Clutch") -> ("error out"=w10:errorcluster, "MotorControlDevRef"=w8:T13)  [unwired: 9 in]
  n188 = call <vilib>:"WPI_MotorControlSetOutput.vi"("error in (no error)"=w10, "Output"=w3, "MotorControlDevRef"=w8) -> ()  [unwired: 6 in, 3 out]
  n189 = call <vilib>:"WPI_MotorControlRefNum Registry Get.vi"("refnum name"="Arm") -> ("MotorControlDevRef"=w57:T13)  [unwired: 9 in, 1 out]
  n190 = call <vilib>:"WPI_MotorControlSetOutput.vi"("Output"=w36, "MotorControlDevRef"=w57) -> ()  [unwired: 7 in, 3 out]
  n191 = disable-structure shown="Disabled" {
    frame Disabled {
      n192 = call <vilib>:"WPI_RelayRefNum Registry Get.vi"("refnum name"="fire") -> ("error out"=w302:errorcluster, "RelayDevRef"=w303:T26)  [unwired: 9 in]
      n193 = call <vilib>:"WPI_RelaySet.vi"("error in (no error)"=w302, "RelayDevRef"=w303) -> ()  [unwired: 8 in, 2 out]
    }
    frame Enabled {
    }
  }
